vi "Write Tx Data (I16).vi"(0 "Register Bus":T1, 5 "data":i16[](array[numeric]), 9 "timeout (s)":dbl=10.0, 11 "error in":errorcluster) -> (4 "Register Bus (out)":T1, 15 "error out":errorcluster)   [LabVIEW 2017]
doc: "Write Tx data to the device. It's required to call <b>Configure Stream</b> and <b>Initiate Stream</b> before calling this VI.\n\n<B>Input Parameters</B>\n\n<B>Register Bus</B> The Register Bus object created by the ni579x Open VI and used as the session handle for the NI-579x Configuration Design Library.\n\n<B>data</B> is the Tx data to write to the device\n\n<B>timeout (s)</B> is how long to wait for (in seconds).\n\n<B>error in</B> describes error conditions that occur before this node runs. This input provides standard 'error in' functionality.\n\n<B>Output Parameters</B>\n\n<B>Register Bus (out)</B> The Register Bus object created by the ni579x Open VI and used as the session handle for the NI-579x Configuration Design Library.\n\n<B>error out</B> contains error information. This output provides standard 'error out' functionality."
uses:
  <instrlib>/_niInstr/Register Bus/v0/Host/Public/Register Bus Session.ctl
  <instrlib>/_niInstr/Register Bus/v0/Host/Private/Session Data.ctl
  Tx FPGA VI Reference.ctl
  <vilib>/Utility/error.llb/Error Cluster From Error Code.vi
  <vilib>/rvi/errors/niLvFpgaAdjustHostInterfaceError.vi
  <vilib>/rvi/interface/nirviMethod/nirviMethod.xnode
  <instrlib>/_niInstr/Register Bus/v0/Host/niInstr Register Bus v0 Host.lvlib
  <vilib>/FPGAPlugInAG/Dynamic/niLvFpga_WriteFifo_Dynamic.vi
  <vilib>/rvi/errors/niLvFpgaMergeErrorWithErrorCode.vi
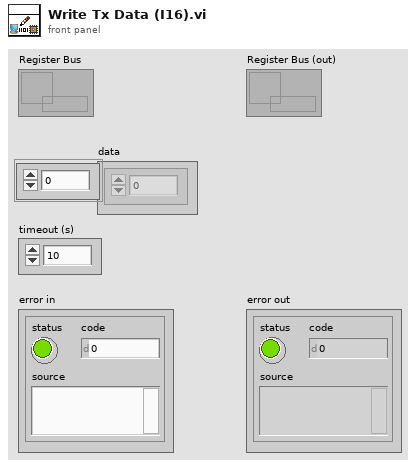
[diagram p1: front panel]
types:
  T1 = typedef "niInstr Register Bus v0 Host.lvlib/Register Bus Session.ctl" = refnum<queue>
  T2 = typedef "Tx FPGA VI Reference.ctl" = refnum<k20>
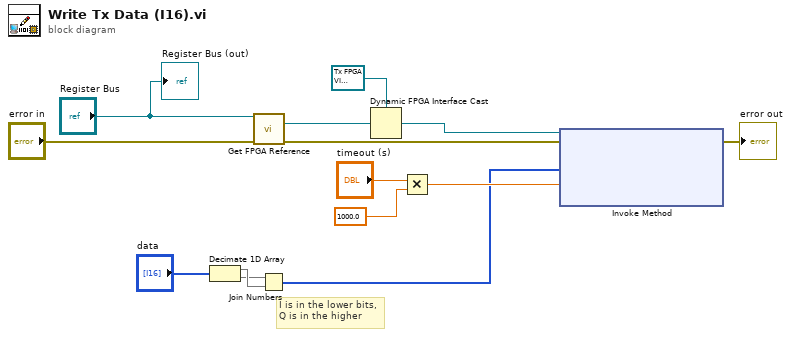
[diagram p0: block diagram]
diagram:
  # "I is in the lower bits,\nQ is in the higher"
  n1 = Decimate 1D Array("data") -> (w2:i16[], w1:i16[])
  n2 = call <instrlib>:"Get FPGA Reference.vi"("session in"="Register Bus", "error in"="error in") -> ("fpga ref"=w11:refnum<k20>, "error out"=w5:errorcluster)  [unwired: 11 in, 1 out]
  n3 = Join Numbers(hi=w1, lo=w2) -> ((hi.lo)=w4:u32[])
  n4 = Dynamic FPGA Interface Cast(Session In=T2 refnum ("Type"), Type=w11) -> (Session Out=w6:T2)
  n5 = Multiply(x="timeout (s)", y=1000.0) -> (x*y=w7:dbl)
  n6 = xnode "Invoke Method"("FPGA VI Reference In"=w6, "error in"=w5, "Data"=w4, "Timeout (ms)"=w7) -> ("error out"=→"error out":errorcluster)  [unwired: 2 out]
  "Register Bus (out)" <- "Register Bus"
